vi "05TRM500_MPHINC_V2.vi"(4 "MPH DOWN":bool, 5 "MPH UP":bool, 6 "INC DOWN":bool, 7 "INC UP":bool, 8 "error in (no error)":errorcluster, 11 "Enum":enum16{"Initialize", "Set"}(ring)) -> (0 "error out":errorcluster, 2 "INC":dbl, 3 "MPH":dbl)   [LabVIEW 2020]
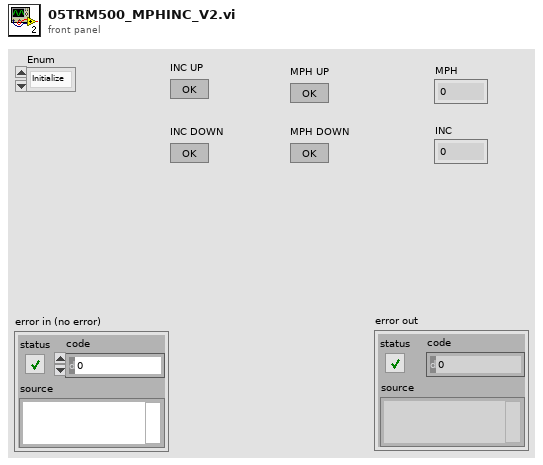
[diagram p1: front panel]
types:
  T1 = enum16{"Initialize", "Next", "Send RSET", "Set MPH", "Set INC", "Part to 0"}
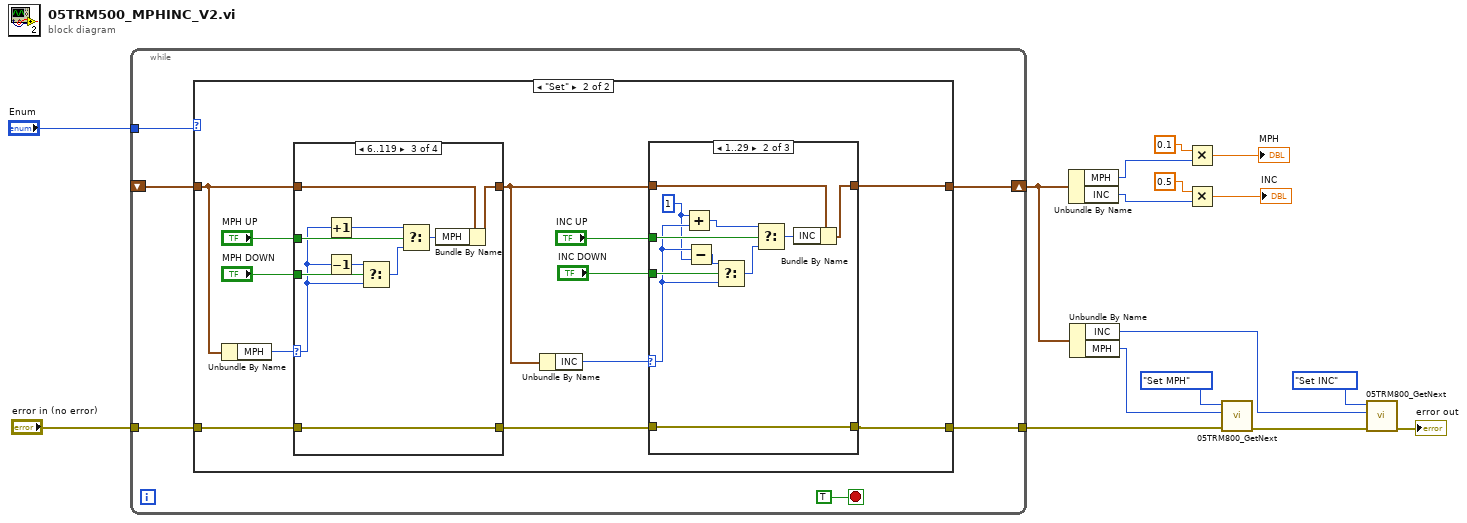
[diagram p0: block diagram]
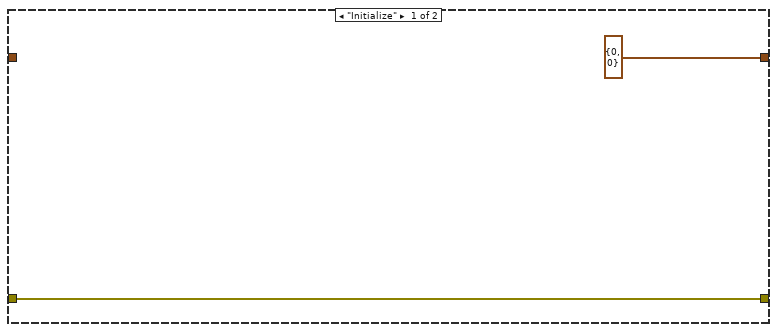
[diagram p2: hidden frame]
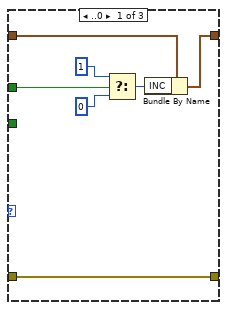
[diagram p3: hidden frame]
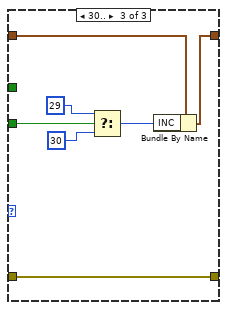
[diagram p4: hidden frame]
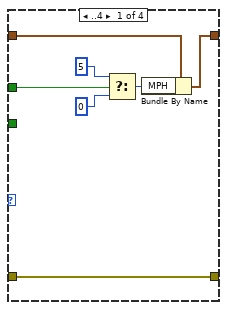
[diagram p5: hidden frame]
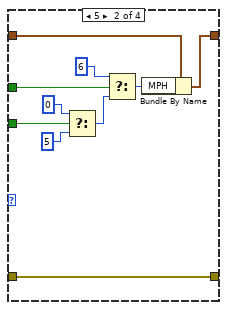
[diagram p6: hidden frame]
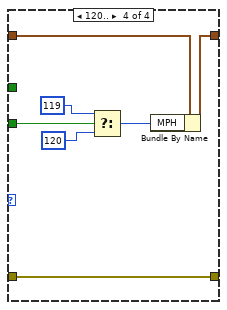
[diagram p7: hidden frame]
diagram:
  n1 = while {
    tunnel: "error in (no error)" -> [w21]
    tunnel: [w20] -> w6
    tunnel: "Enum" -> [w19]
    shift-right: [w18] -> w9
    shift-left: _ -> [w17]
    stop <- TRUE stop-if-true
    n2 = case shown="\"Set\"" w19 {
      tunnel: w21 -> [w24 w36]
      tunnel: [w24 w27] -> w20
      tunnel: [cluster{"MPH":i32, "INC":i32} {"MPH"=0, "INC"=0} w26] -> w18
      tunnel: w17 -> [_ w34]
      frame "Initialize" {
      }
      frame "Set" {
        n3 = Unbundle By Name(w34) -> ("MPH"=w35:i32)
        n4 = case shown="6..119" w35 {
          selector: w35 -> [_ _ w80 _]
          tunnel: w36 -> [w68 w78 w88 w95]
          tunnel: [w68 w78 w88 w95] -> w31
          tunnel: w34 -> [w66 w76 w86 w93]
          tunnel: "MPH UP" -> [w65 w75 w85 _]
          tunnel: "MPH DOWN" -> [_ w71 w82 w92]
          tunnel: [w67 w77 w87 w94] -> w30
          frame ..4 {
            n5 = Select(t=5 ("MPH"), s=w65, f=0 ("MPH")) -> (s? t:f=w64:i32)
            n6 = Bundle By Name(cluster=w66, "MPH"=w64) -> (w67:cluster{"MPH":i32, "INC":i32})
          }
          frame 5 {
            n7 = Select(t=0 ("MPH"), s=w71, f=5 ("MPH")) -> (s? t:f=w72:i32)
            n8 = Select(t=6 ("MPH"), s=w75, f=w72) -> (s? t:f=w74:i32)
            n9 = Bundle By Name(cluster=w76, "MPH"=w74) -> (w77:cluster{"MPH":i32, "INC":i32})
          }
          frame 6..119 {
            n10 = Increment(x=w80) -> (x+1=w79:i32)
            n11 = Decrement(x=w80) -> (x-1=w81:i32)
            n12 = Select(t=w81, s=w82, f=w80) -> (s? t:f=w83:i32)
            n13 = Select(t=w79, s=w85, f=w83) -> (s? t:f=w84:i32)
            n14 = Bundle By Name(cluster=w86, "MPH"=w84) -> (w87:cluster{"MPH":i32, "INC":i32})
          }
          frame 120.. {
            n15 = Select(t=119 ("MPH"), s=w92, f=120) -> (s? t:f=w91:i32)
            n16 = Bundle By Name(cluster=w93, "MPH"=w91) -> (w94:cluster{"MPH":i32, "INC":i32})
          }
        }
        n17 = Unbundle By Name(w30) -> ("INC"=w25:i32)
        n18 = case shown="1..29" w25 {
          selector: w25 -> [_ w46 _]
          tunnel: w31 -> [w43 w54 w61]
          tunnel: [w43 w54 w61] -> w27
          tunnel: w30 -> [w41 w52 w59]
          tunnel: "INC UP" -> [w40 w51 _]
          tunnel: "INC DOWN" -> [_ w48 w58]
          tunnel: [w42 w53 w60] -> w26
          frame ..0 {
            n19 = Select(t=1 ("MPH"), s=w40, f=0 ("MPH")) -> (s? t:f=w39:i32)
            n20 = Bundle By Name(cluster=w41, "INC"=w39) -> (w42:cluster{"MPH":i32, "INC":i32})
          }
          frame 1..29 {
            w45 = 1
            n21 = Add(x=w45, y=w46) -> (x+y=w47:i32)
            n22 = Subtract(x=w46, y=w45) -> (x-y=w44:i32)
            n23 = Select(t=w44, s=w48, f=w46) -> (s? t:f=w49:i32)
            n24 = Select(t=w47, s=w51, f=w49) -> (s? t:f=w50:i32)
            n25 = Bundle By Name(cluster=w52, "INC"=w50) -> (w53:cluster{"MPH":i32, "INC":i32})
          }
          frame 30.. {
            n26 = Select(t=29 ("MPH"), s=w58, f=30) -> (s? t:f=w57:i32)
            n27 = Bundle By Name(cluster=w59, "INC"=w57) -> (w60:cluster{"MPH":i32, "INC":i32})
          }
        }
      }
    }
  }
  n28 = Unbundle By Name(w9) -> ("MPH"=w14:i32, "INC"=w11:i32)
  n29 = Unbundle By Name(w9) -> ("INC"=w2:i32, "MPH"=w7:i32)
  n30 = Multiply(x=0.1, y=w14) -> (x*y=→"MPH":dbl)
  n31 = Multiply(x=0.5, y=w11) -> (x*y=→"INC":dbl)
  n32 = call "05TRM800_GetNext.vi"("error in (no error)"=w6, "Value"=w7, "Enum"=T1."Set MPH") -> ("error out"=w3:errorcluster)  [unwired: 7 in, 1 out]
  n33 = call "05TRM800_GetNext.vi"("error in (no error)"=w3, "Value"=w2, "Enum"=T1."Set INC") -> ("error out"=→"error out":errorcluster)  [unwired: 7 in, 1 out]
